vi "Draw Robot XY Graph.vi"(11 "Pose":cluster{"x":dbl, "y":dbl, "theta":dbl}) -> (3 "Robot Pose":cluster{cluster{dbl, dbl}[]}[](graph))   [LabVIEW 2023]
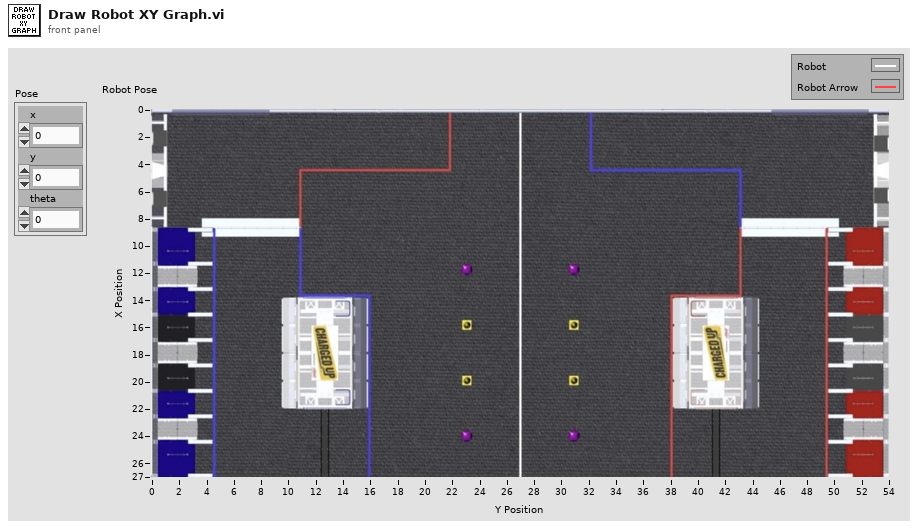
[diagram p1: front panel]
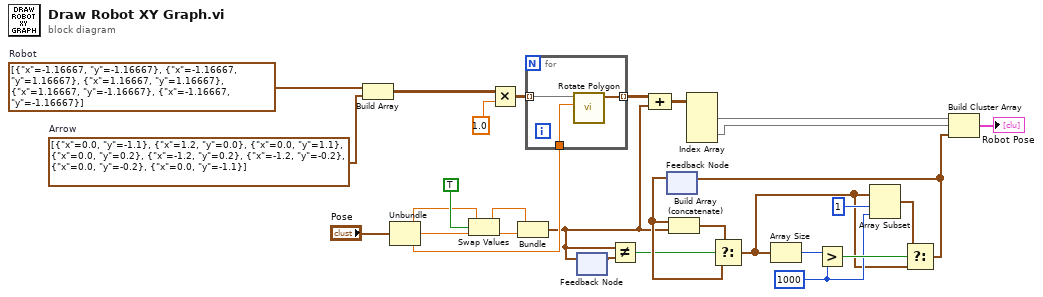
[diagram p0: block diagram]
diagram:
  w9 = 1000 ("y")
  w27 = cluster{"x":dbl, "y":dbl}[] [{"x"=-1.16667, "y"=-1.16667}, {"x"=-1.16667, "y"=1.16667}, {"x"=1.16667, "y"=1.16667}, {"x"=1.16667, "y"=-1.16667}, {"x"=-1.16667, "y"=-1.16667}]  # Robot
  w26 = cluster{"x":dbl, "y":dbl}[] [{"x"=0.0, "y"=-1.1}, {"x"=1.2, "y"=0.0}, {"x"=0.0, "y"=1.1}, {"x"=0.0, "y"=0.2}, {"x"=-1.2, "y"=0.2}, {"x"=-1.2, "y"=-0.2}, {"x"=0.0, "y"=-0.2}, {"x"=0.0, "y"=-1.1}]  # Arrow
  n1 = Build Array(w27, w26) -> (w25:cluster{"x":dbl, "y":dbl}[][])
  n2 = Unbundle("Pose") -> ("x"=w13:dbl, "y"=w18:dbl, "theta"=w14:dbl)
  n3 = Swap Values(12:w13, 13:TRUE ("?(T)"), 14:w18) -> (1:w16:dbl, 3:w15:dbl)
  n4 = Multiply(x=w25, y=1.0 ("Scale")) -> (x*y=w28:cluster{"x":dbl, "y":dbl}[][])
  n5 = Bundle(w16, w15) -> (w2:cluster{dbl, dbl})  [unwired: 1 in]
  n6 = for {
    tunnel: w14 -> [w30]
    tunnel: [w31] -> w24 mode=indexing
    tunnel: w28 -> [w32] mode=indexing
    n7 = call "Rotate Polygon.vi"("Angle"=w30, "Input Polygon"=w32) -> ("Output Polygon"=w31:cluster{dbl, dbl}[])  [unwired: 9 in]
  }
  n8 = feedback-in #1(w2) -> ()
  n9 = feedback #1() -> (w3:cluster{dbl, dbl})  [unwired: 1 in]
  n10 = Not Equal?(x=w2, y=w3) -> (x != y?=w1:bool)
  n11 = Compound Arithmetic op=ADD(w24, w2) -> (w23:cluster{dbl, dbl}[][])
  n12 = feedback #2() -> (w5:cluster{dbl, dbl}[])  [unwired: 1 in]
  n13 = Build Array (concatenate)(w5, w2) -> (w6:cluster{dbl, dbl}[])
  n14 = Index Array(array=w23) -> (element #1=w21:cluster{dbl, dbl}[], element #2=w20:cluster{dbl, dbl}[])  [unwired: 4 in]
  n15 = Select(t=w6, s=w1, f=w5) -> (s? t:f=w4:cluster{dbl, dbl}[])
  n16 = Array Size(array=w4) -> (size(s)=w12:i32)
  n17 = Greater?(x=w12, y=w9) -> (0:w11:bool)
  n18 = Array Subset(array=w4, index=1, length=w9) -> (w10:cluster{dbl, dbl}[])
  n19 = Select(t=w10, s=w11, f=w4) -> (s? t:f=w7:cluster{dbl, dbl}[])
  n20 = feedback-in #2(w7) -> ()
  n21 = Build Cluster Array(w21, w20, w7) -> (→"Robot Pose":cluster{cluster{dbl, dbl}[]}[])
